vi "Complex Matrix Square Root.vi"(3 "Input Matrix":T1) -> (0 "error":i32, 1 "Matrix Square Root":T1)   [LabVIEW 2017, in "NI_AALBase.lvlib"]
doc: "Computes the square root of <B>Input Matrix</B>. Wire data to the <B>Input Matrix</B> input to determine the polymorphic instance to use or manually select the instance."
uses:
  NI_AALBase.lvlib
  ComplexMatrix.ctl
  <resource>/lvanlys.dll
  NI_Matrix.lvlib
panel:
  # "Complex Matrix Square Root"
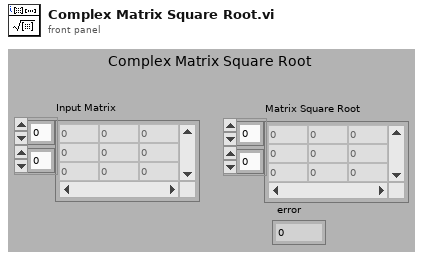
[diagram p1: front panel]
types:
  T1 = typedef "NI_Matrix.lvlib/ComplexMatrix.ctl" = cdb[][]
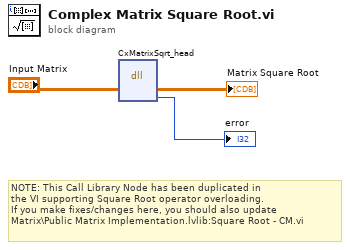
[diagram p0: block diagram]
diagram:
  # "NOTE: This Call Library Node has been duplicated in\nthe VI supporting Square Root operator overloading.\nIf you make fixes/changes here, you should also update\nMatrix\\Public Matrix Implementation.lvlib:Square Root - CM.vi"
  n1 = dll-call lib="C:/Program Files (x86)/National Instruments/LabVIEW 2017/resource/lvanlys.*" fn="CxMatrixSqrt_head"("Input Matrix"="Input Matrix") -> ("Input Matrix"=→"Matrix Square Root":T1, "error"=→"error":i32)  [unwired: 5 in, 2 out]
